vi "Set_RAW.vi"(0 "reference in":refnum<class "Sig_AI.lvclass">, 5 "RAW":dbl, 11 "error in (no error)":errorcluster) -> (4 "reference out":refnum<class "Sig_AI.lvclass">, 15 "error out":errorcluster)   [LabVIEW 2019, in "Sig_AI.lvclass"]
uses:
  Sig_AI.lvclass
  D:/H4000/src/Proccess_class/Proccess.lvclass
  Sig_AI.lvclass/Sig_AI.ctl
  Proccess_class/Proccess.lvclass/Proccess.ctl
  Logger_class/Logger.lvclass/Logger.ctl
  AnalogComparator_class/AnalogComparator.lvclass/AnalogComparator.ctl
  Logger_class/Enqueue Signal.vi
  Proccess_class/Read TagName.vi
  Proccess_class/Read Logger.vi
  AnalogComparator_class/SetValue.vi
  AnalogComparator_class/HandleDb.vi
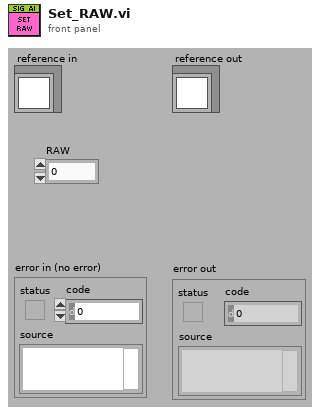
[diagram p1: front panel]
types:
  T1 = typedef "Config_Scale.ctl" = cluster{"scale [EU/RAW]":dbl, "offset [EU]":dbl}
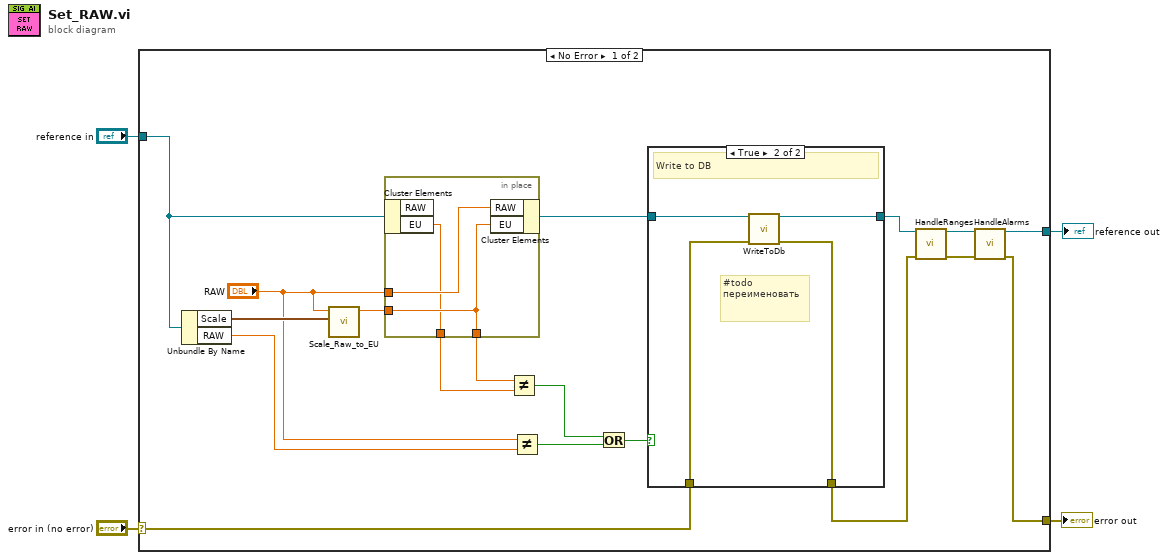
[diagram p0: block diagram]
diagram:
  n1 = case shown="No Error" "error in (no error)" {
    selector: "error in (no error)" -> [w22 w33]
    tunnel: [w10 w33] -> w3
    tunnel: [w11 w32] -> w1
    tunnel: "reference in" -> [w17 w32]
    frame No Error {
      n2 = Unbundle By Name(w17) -> ("Scale"=w21:T1, "RAW"=w19:dbl)
      n3 = call "Scale_Raw_to_EU.vi"("ConfigScale"=w21, "RAW"="RAW") -> ("EU"=w9:dbl)  [unwired: 9 in]
      n4 = in-place {
        in-place-border: "RAW" -> [w31]
        in-place-border: w9 -> [w30]
        in-place-border: [w30] -> w8
        in-place-border: [w29] -> w7
        n5 = in-place-cluster #1(w17) -> ("EU"=w29:dbl)  [unwired: 1 out]
        n6 = in-place-cluster #1("RAW"=w31, "EU"=w30) -> (w16:refnum<class "Sig_AI.lvclass">)
      }
      n7 = Not Equal?(x=w8, y=w7) -> (x != y?=w5:bool)
      n8 = Not Equal?(x="RAW", y=w19) -> (x != y?=w18:bool)
      n9 = Or(x=w5, y=w18) -> (x .or. y?=w6:bool)
      n10 = case shown="True" w6 {
        tunnel: w16 -> [w24 w28]
        tunnel: [w24 w27] -> w15
        tunnel: [w23 w25] -> w14
        tunnel: w22 -> [w23 w26]
        frame False {
        }
        frame True {
          # "#todo\nпереименовать"
          # "Write to DB"
          n11 = call "WriteToDb.vi"("reference in"=w28, "error in (no error)"=w26) -> ("reference out"=w27:refnum<class "Sig_AI.lvclass">, "error out"=w25:errorcluster)  [unwired: 12 in]
        }
      }
      n12 = call "HandleRanges.vi"("reference in"=w15, "error in (no error)"=w14) -> ("reference out"=w13:refnum<class "Sig_AI.lvclass">, "error out"=w12:errorcluster)  [unwired: 12 in]
      n13 = call "HandleAlarms.vi"("reference in"=w13, "error in (no error)"=w12) -> ("reference out"=w11:refnum<class "Sig_AI.lvclass">, "error out"=w10:errorcluster)  [unwired: 12 in]
    }
    frame Error {
    }
  }
  "error out" <- w3
  "reference out" <- w1
